vi "LCS kNN.vi"() -> ()   [LabVIEW 2014]
panel:
  out "subarray":dbl[](array[numeric])
  out "size(s) 2":i32
  out "size(s)":i32
  out "accuracy":string[][](array[string])
  out "Results":string[][](array[string])
  out "Array":string[][](array[string])
  in  "kNN k":i32=5
  out "appended array":string[](array[string])
  out "Numeric":i32
  in  "all rows":string[][](array[string])=array2038x3[6114 elements]
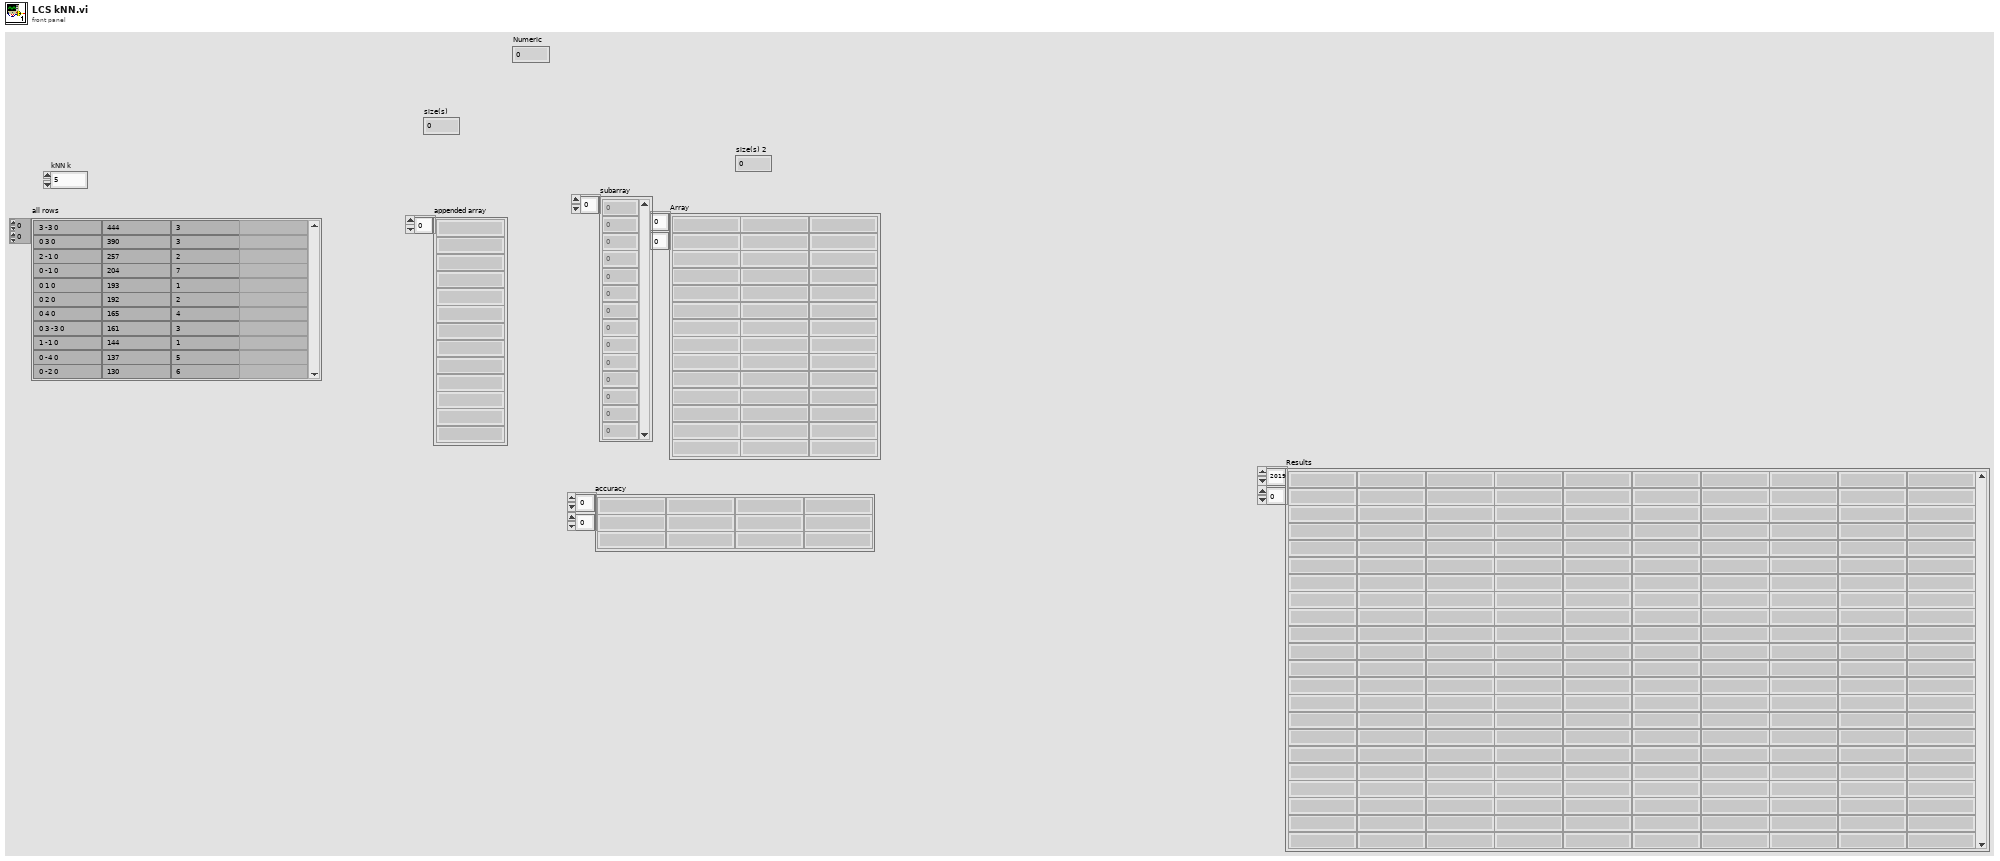
[diagram p1: front panel]
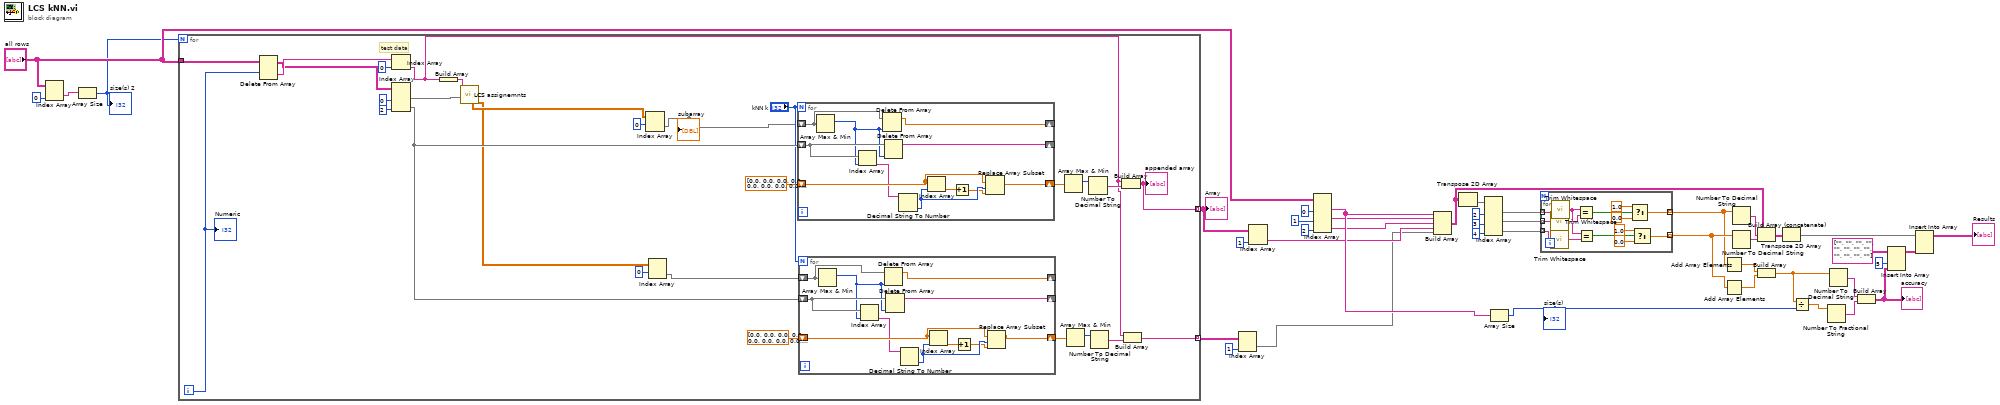
[diagram p0: block diagram]
diagram:
  n1 = Index Array(array="all rows", index (col)=0 ("disabled index (col)")) -> (element=w2:string[])  [unwired: 1 in]
  n2 = Array Size(array=w2) -> (size(s)=w1:i32)
  "size(s) 2" <- w1
  n3 = for {
    N: w1 -> [_]
    tunnel: "all rows" -> [w70]
    tunnel: [w59] -> w9 mode=indexing
    tunnel: [w52] -> w6 mode=indexing
    i -> [w69]
    # "test data"
    n4 = Delete From Array(array=w70, index (row)=w69) -> (deleted portion=w68:string[], array with subset deleted=w65:string[][])  [unwired: 2 in]
    n5 = Index Array(array=w68, index=0 ("disabled index (col)")) -> (element=w53:string)
    n6 = Index Array(array=w65, index (col) #1=0 ("disabled index (col)"), index (col) #2=2 ("index (col)")) -> (element #1=w49:string[], element #2=w54:string[])  [unwired: 2 in]
    n7 = Build Array(w53) -> (w50:string[])
    n8 = call "LCS assignemnts.vi"("cluster centers"=w49, "Patterns in"=w50) -> ("LCS/Lsample (zeroed)/Lknown"=w43:dbl[][], "Distance values (LCS)"=w44:dbl[][])  [unwired: 3 in, 5 out]
    n9 = Index Array(array=w44, index (row)=0) -> (element=w47:dbl[])  [unwired: 1 in]
    "subarray" <- w47
    n10 = Index Array(array=w43, index (row)=0) -> (element=w45:dbl[])  [unwired: 1 in]
    n11 = for {
      N: "kNN k" -> [_]
      shift-right: [w89] -> _
      shift-left: w47 -> [w92]
      shift-right: [w88] -> _
      shift-left: w54 -> [w91]
      shift-right: [w83] -> w62
      shift-left: dbl[] [0.0, 0.0, 0.0, 0.0, 0.0, 0.0, 0.0, 0.0, 0.0, 0.0, 0.0, 0.0] -> [w84]
      n12 = Array Max & Min(array=w92) -> (max index (indices)=w90:i32)  [unwired: 3 out]
      n13 = Index Array(array=w91, index=w90) -> (element=w82:string)
      n14 = Delete From Array(array=w92, index=w90) -> (array with subset deleted=w89:dbl[])  [unwired: 1 in, 1 out]
      n15 = Delete From Array(array=w91, index=w90) -> (array with subset deleted=w88:string[])  [unwired: 1 in, 1 out]
      n16 = Decimal String To Number(string=w82) -> (number=w87:i32)  [unwired: 2 in, 1 out]
      n17 = Index Array(array=w84, index=w87) -> (element=w85:dbl)
      n18 = Increment(x=w85) -> (x+1=w86:dbl)
      n19 = Replace Array Subset(array=w84, new element=w86, index=w87) -> (w83:dbl[])
    }
    n20 = for {
      N: "kNN k" -> [_]
      shift-right: [w71] -> _
      shift-left: w45 -> [w72]
      shift-right: [w79] -> _
      shift-left: w54 -> [w81]
      shift-right: [w74] -> w56
      shift-left: dbl[] [0.0, 0.0, 0.0, 0.0, 0.0, 0.0, 0.0, 0.0, 0.0, 0.0, 0.0, 0.0] -> [w75]
      n21 = Array Max & Min(array=w72) -> (max index (indices)=w80:i32)  [unwired: 3 out]
      n22 = Index Array(array=w81, index=w80) -> (element=w73:string)
      n23 = Delete From Array(array=w72, index=w80) -> (array with subset deleted=w71:dbl[])  [unwired: 1 in, 1 out]
      n24 = Delete From Array(array=w81, index=w80) -> (array with subset deleted=w79:string[])  [unwired: 1 in, 1 out]
      n25 = Decimal String To Number(string=w73) -> (number=w78:i32)  [unwired: 2 in, 1 out]
      n26 = Index Array(array=w75, index=w78) -> (element=w76:dbl)
      n27 = Increment(x=w76) -> (x+1=w77:dbl)
      n28 = Replace Array Subset(array=w75, new element=w77, index=w78) -> (w74:dbl[])
    }
    n29 = Array Max & Min(array=w62) -> (max index (indices)=w61:i32)  [unwired: 3 out]
    n30 = Array Max & Min(array=w56) -> (max index (indices)=w57:i32)  [unwired: 3 out]
    n31 = Number To Decimal String(number=w61) -> (decimal integer string=w63:string)  [unwired: 1 in]
    n32 = Number To Decimal String(number=w57) -> (decimal integer string=w55:string)  [unwired: 1 in]
    n33 = Build Array(w53, w63) -> (w59:string[])
    "appended array" <- w59
    n34 = Build Array(w53, w55) -> (w52:string[])
    "Numeric" <- w69
  }
  "Array" <- w9
  n35 = Index Array(array=w6, index (col)=1 ("disabled index (col)")) -> (element=w5:string[])  [unwired: 1 in]
  n36 = Index Array(array=w9, index (col)=1 ("disabled index (col)")) -> (element=w8:string[])  [unwired: 1 in]
  n37 = Index Array(array="all rows", index (col) #1=0 ("disabled index (col)"), index (col) #2=1 ("index (col)"), index (col) #3=2 ("index (col)")) -> (element #1=w41:string[], element #2=w37:string[], element #3=w38:string[])  [unwired: 3 in]
  n38 = Build Array(w41, w37, w38, w8, w5) -> (w40:string[][])
  n39 = Transpose 2D Array(2D array=w40) -> (transposed array=w19:string[][])
  n40 = Index Array(array=w19, index (col) #1=2 ("disabled index (col)"), index (col) #2=3 ("index (col)"), index (col) #3=4 ("index (col)")) -> (element #1=w16:string[], element #2=w17:string[], element #3=w18:string[])  [unwired: 3 in]
  n41 = Array Size(array=w41) -> (size(s)=w42:i32)
  "size(s)" <- w42
  n42 = for {
    tunnel: w16 -> [w98] mode=indexing
    tunnel: w17 -> [w97] mode=indexing
    tunnel: w18 -> [w96] mode=indexing
    tunnel: [w100] -> w34 mode=indexing
    tunnel: [w99] -> w35 mode=indexing
    n43 = call <vilib>:"Trim Whitespace.vi"("string"=w97) -> ("trimmed string"=w95:string)  [unwired: 1 in]
    n44 = call <vilib>:"Trim Whitespace.vi"("string"=w96) -> ("trimmed string"=w94:string)  [unwired: 1 in]
    n45 = call <vilib>:"Trim Whitespace.vi"("string"=w98) -> ("trimmed string"=w93:string)  [unwired: 1 in]
    n46 = Equal?(x=w93, y=w95) -> (x = y?=w106:bool)
    n47 = Equal?(x=w93, y=w94) -> (x = y?=w101:bool)
    n48 = Select(t=1.0, s=w106, f=0.0) -> (s? t:f=w100:dbl)
    n49 = Select(t=1.0, s=w101, f=0.0) -> (s? t:f=w99:dbl)
  }
  n50 = Add Array Elements(numeric array=w34) -> (sum=w33:dbl)
  n51 = Add Array Elements(numeric array=w35) -> (sum=w32:dbl)
  n52 = Number To Decimal String(number=w34) -> (decimal integer string=w20:string[])  [unwired: 1 in]
  n53 = Number To Decimal String(number=w35) -> (decimal integer string=w21:string[])  [unwired: 1 in]
  n54 = Build Array (concatenate)(w40, w20, w21) -> (w22:string[][])
  n55 = Build Array(w33, w32) -> (w31:dbl[])
  n56 = Transpose 2D Array(2D array=w22) -> (transposed array=w36:string[][])
  n57 = Divide(x=w31, y=w42) -> (x/y=w30:dbl[])
  n58 = Number To Fractional String(number=w30) -> (F-format string=w28:string[])  [unwired: 3 in]
  n59 = Number To Decimal String(number=w31) -> (decimal integer string=w29:string[])  [unwired: 1 in]
  n60 = Build Array(w29, w28) -> (w24:string[][])
  "accuracy" <- w24
  n61 = Insert Into Array(array=string[][] [["", "", "", "", "", ""], ["", "", "", "", "", ""]] ("appended array 3"), index (col)=5 ("disabled index (col)"), new element=w24) -> (w25:string[][])  [unwired: 1 in]
  n62 = Insert Into Array(array=w36, new element=w25) -> (→"Results":string[][])  [unwired: 2 in]
